vi "ArdnoManualValvesFromUI.vi"(8 "error in (no error)":errorcluster, 10 "LINX Resource":T1, 11 "reference":refnum<vi>) -> (0 "error out":errorcluster)   [LabVIEW 2018]
uses:
  <vilib>/MakerHub/LINX/Private/Type Defs/LINX Ref.ctl
  <vilib>/MakerHub/LINX/Private/Type Defs/Platform.ctl
  <vilib>/MakerHub/LINX/Private/Type Defs/Interface.ctl
  <vilib>/MakerHub/LINX/Private/Device/Type Defs/LINX Device Config.ctl
  <vilib>/MakerHub/LINX/Private/Device/Type Defs/TCP Config.ctl
  <vilib>/MakerHub/LINX/Private/Device/Type Defs/Channels.ctl
  <vilib>/MakerHub/LINX/Public/Peripherals/Digital/Digital Write N Chans.vi
  <vilib>/MakerHub/LINX/Private/Local IO/LinxDigitalWrite.vi
  <vilib>/MakerHub/LINX/Public/Utilities/Check Channel.vi
  <vilib>/MakerHub/LINX/Private/Utilties/Generate Error.vi
  <vilib>/MakerHub/LINX/LMH-LINX.lvlib
  <vilib>/MakerHub/LINX/Private/Device/Device.lvlib
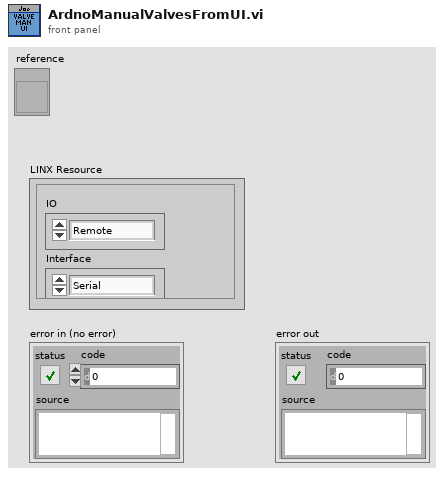
[diagram p1: front panel]
types:
  T1 = typedef "LMH-LINX.lvlib/LINX Ref.ctl" = cluster{"IO":T2, "Interface":T3, "LINX Device Config":T4}
  T2 = typedef "LMH-LINX.lvlib/Platform.ctl" = enum16{"Remote", "Local"}
  T3 = typedef "LMH-LINX.lvlib/Interface.ctl" = enum16{"Serial", "TCP"}
  T4 = typedef "LMH-LINX.lvlib/Device.lvlib/LINX Device Config.ctl" = cluster{"Interface":T3, "COM Port":refnum<visa-resource-name>, "TCP Configuration":T5, "Device Family":u8, "Device ID":u8, "Device Name":string, "TCP Ref":refnum<k5>, "Channels":T6}
  T5 = typedef "LMH-LINX.lvlib/Device.lvlib/TCP Config.ctl" = cluster{"IP Address":string, "Port":u16}
  T6 = typedef "LMH-LINX.lvlib/Channels.ctl" = cluster{"DI":u8[], "DO":u8[], "AI":u8[], "AO":u8[], "PWM":u8[], "QE":u8[], "UART":u8[], "I2C 2":u8[], "SPI":u8[], "CAN":u8[], "Servo":u8[], "AI Ref (V)":dbl, "AI Resolution (Bits)":u8, "AO Ref (V)":dbl, "AO Resolution (Bits)":u8}
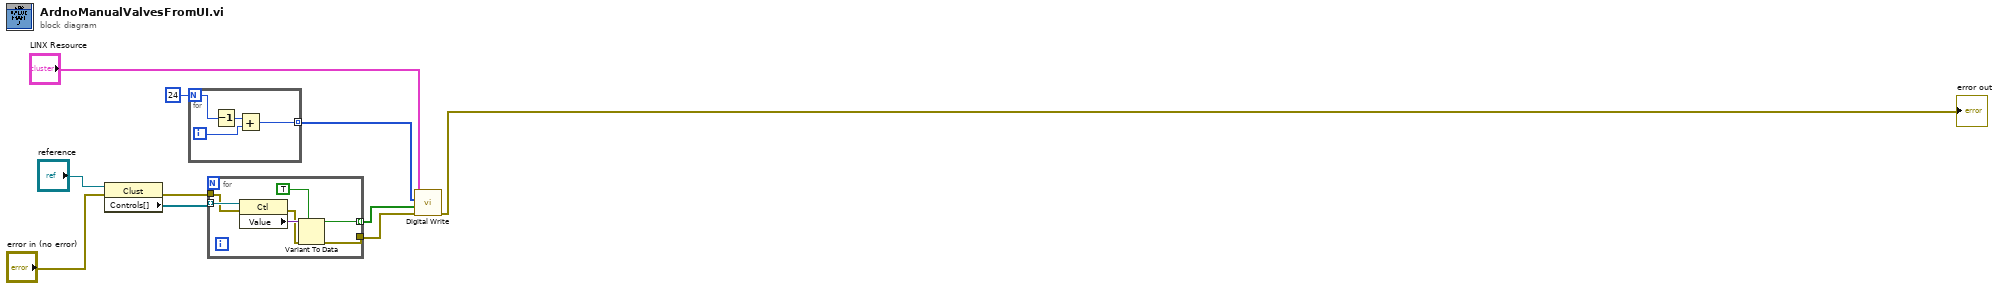
[diagram p0: block diagram]
diagram:
  n1 = property class="Clust"(reference="reference", error in="error in (no error)") -> (error out=w4:errorcluster, "Controls[]"=w2:refnum<vi>[])  [unwired: 1 out]
  n2 = for {
    N: 24 -> [w14]
    tunnel: [w11] -> w9 mode=indexing
    i -> [w12]
    n3 = Decrement(x=w14) -> (x-1=w13:i32)
    n4 = Add(x=w13, y=w12) -> (x+y=w11:i32)
  }
  n5 = for {
    tunnel: w2 -> [w21] mode=indexing
    tunnel: [w19] -> w8 mode=indexing
    tunnel: [w16] -> w7
    tunnel: w4 -> [w15]
    n6 = property class="Ctl"(reference=w21, error in=w15) -> (error out=w17:errorcluster, "Value"=w20:variant)  [unwired: 1 out]
    n7 = Variant To Data(error in=w17, type=TRUE, Variant=w20) -> (data=w19:bool, error out=w16:errorcluster)
  }
  n8 = call-poly <vilib>:"Digital Write.vi"("Error In"=w7, "Values"=w8, "DO Channels"=w9, "LINX Resource"="LINX Resource") -> ("Error Out"=→"error out":errorcluster)  [unwired: 6 in, 1 out]
